vi "Estimate Mecanum Steering Frame.vi"(8 "error in (no error)":errorcluster, 11 "steering frame in":refnum<class "NI_Robotics_Steering Frame.lvclass">) -> (0 "error out":errorcluster, 2 "estimated mecanum steering frame copy":refnum<class "NI_Robotics_Mecanum Steering Frame.lvclass">, 3 "steering frame out":refnum<class "NI_Robotics_Steering Frame.lvclass">)   [LabVIEW 2017, in "NI_Robotics_Configure Steering Frame.lvlib"]
uses:
  <vilib>/robotics/Dialog/Configure Steering Frame/NI_Robotics_Configure Steering Frame.lvlib
  <vilib>/robotics/Steering/Steering Frame/NI_Robotics_Steering Frame.lvclass
  <vilib>/robotics/Steering/Mecanum Steering Frame/NI_Robotics_Mecanum Steering Frame.lvclass
  <vilib>/robotics/Steering/Steering Frame/NI_Robotics_Steering Frame.lvclass/NI_Robotics_Steering Frame.ctl
  <vilib>/robotics/Steering/Wheel/Wheel Parameters.ctl
  <vilib>/robotics/Steering/Wheel/Rotation Direction.ctl
  <vilib>/robotics/Steering/Mecanum Wheel/NI_Robotics_Mecanum Wheel.lvclass
  c:/Program Files (x86)/National Instruments/LabVIEW 2017/vi.lib/robotics/Steering/Wheel/NI_Robotics_Wheel.lvclass
  <vilib>/robotics/Steering/Wheel/NI_Robotics_Wheel.lvclass/NI_Robotics_Wheel.ctl
  <vilib>/robotics/Steering/Steering Frame/Get Multiple Wheels in Steering Frame.vi
  <vilib>/robotics/Steering/Wheel/Get General Wheel Information.vi
  <vilib>/robotics/Steering/Wheel/Get Wheel Radius.vi
  <vilib>/robotics/Steering/Wheel/Get Motor Communication.vi
  <vilib>/robotics/Steering/Wheel/Get Wheel Parameters.vi
  <vilib>/robotics/Steering/Mecanum Steering Frame/Create Mecanum Steering Frame.vi
  <vilib>/robotics/Steering/Omnidirectional Wheel/Create Omnidirectional Wheel.vi
  <vilib>/robotics/Steering/Mecanum Wheel/Create Mecanum Wheel.vi
  <vilib>/robotics/Steering/Caster Wheel/Create Caster Wheel.vi
  <vilib>/robotics/Steering/Steering Wheel/Create Steering Wheel.vi
  <vilib>/robotics/Steering/Fixed Wheel/Create Fixed Wheel.vi
  <vilib>/robotics/Steering/Wheel/NI_Robotics_Wheel.lvclass
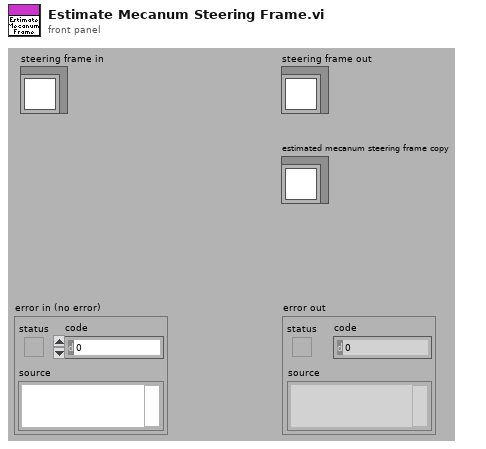
[diagram p1: front panel]
types:
  T1 = typedef "NI_Robotics_Wheel.lvclass/Wheel Parameters.ctl" = cluster{"wheel radius":dbl, "gear ratio":dbl, "forward rotation direction":T2}
  T2 = typedef "NI_Robotics_Wheel.lvclass/Rotation Direction.ctl" = u16
  T3 = cluster{"[0]":refnum<class "NI_Robotics_Mecanum Wheel.lvclass">, "[1]":refnum<class "NI_Robotics_Mecanum Wheel.lvclass">, "[2]":refnum<class "NI_Robotics_Mecanum Wheel.lvclass">, "[3]":refnum<class "NI_Robotics_Mecanum Wheel.lvclass">}
  T4 = cluster{"NI_Robotics_Mecanum Wheel.lvclass":refnum<class "NI_Robotics_Mecanum Wheel.lvclass">, "NI_Robotics_Mecanum Wheel.lvclass":refnum<class "NI_Robotics_Mecanum Wheel.lvclass">, "NI_Robotics_Mecanum Wheel.lvclass":refnum<class "NI_Robotics_Mecanum Wheel.lvclass">, "NI_Robotics_Mecanum Wheel.lvclass":refnum<class "NI_Robotics_Mecanum Wheel.lvclass">}
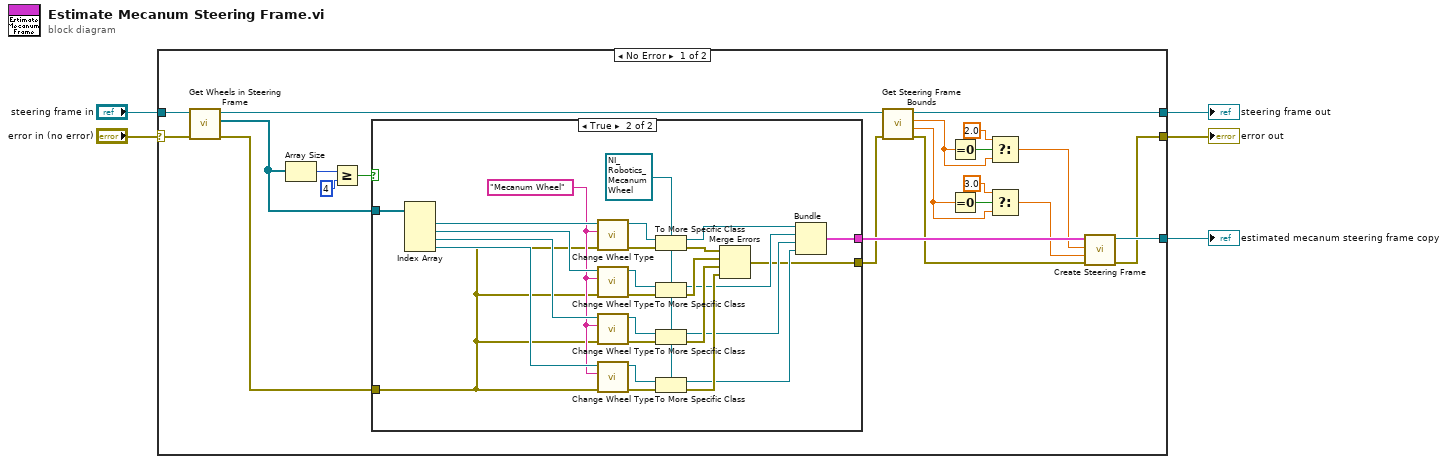
[diagram p0: block diagram]
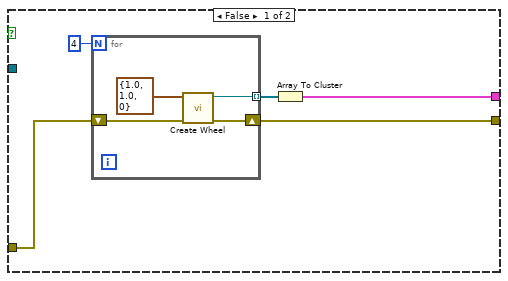
[diagram p2: hidden frame]
diagram:
  n1 = case shown="No Error" "error in (no error)" {
    selector: "error in (no error)" -> [w27 w64]
    tunnel: [w24 w64] -> w4
    tunnel: "steering frame in" -> [w26 w63]
    tunnel: [w17 w63] -> w2
    tunnel: [w25 _] -> w1
    frame No Error {
      n2 = call-poly <vilib>:"Get Wheels in Steering Frame.vi"("error in (no error)"=w27, "steering frame in"=w26) -> ("error out"=w19:errorcluster, "wheels"=w20:refnum<class "NI_Robotics_Wheel.lvclass">[], "steering frame out"=w6:refnum<class "NI_Robotics_Steering Frame.lvclass">)  [unwired: 3 in, 4 out]
      n3 = Array Size(array=w20) -> (size(s)=w23:i32)
      n4 = Greater Or Equal?(x=w23, y=4) -> (x >= y?=w21:bool)
      n5 = case shown="True" w21 {
        tunnel: w20 -> [_ w60]
        tunnel: w19 -> [w30 w37]
        tunnel: [w28 w41] -> w18
        tunnel: [w32 w40] -> w7
        frame False {
          n6 = for {
            N: 4 -> [_]
            shift-right: [w35] -> w32
            shift-left: w30 -> [w36]
            tunnel: [w34] -> w29 mode=indexing
            n7 = call-poly <vilib>:"Create Wheel.vi"("error in (no error)"=w36, "wheel parameters"=T1 {"wheel radius"=1.0, "gear ratio"=1.0, "forward rotation direction"=0}) -> ("error out"=w35:errorcluster, "mecanum wheel out"=w34:refnum<class "NI_Robotics_Mecanum Wheel.lvclass">)  [unwired: 8 in]
          }
          n8 = Array To Cluster(array=w29) -> (cluster=w28:T3)
        }
        frame True {
          w38 = refnum<class "NI_Robotics_Mecanum Wheel.lvclass"> refnum ("NI_Robotics_Mecanum Wheel.lvclass")
          w39 = "Mecanum Wheel" ("wheel type")
          n9 = Index Array(array=w60) -> (element #1=w59:refnum<class "NI_Robotics_Wheel.lvclass">, element #2=w55:refnum<class "NI_Robotics_Wheel.lvclass">, element #3=w54:refnum<class "NI_Robotics_Wheel.lvclass">, element #4=w53:refnum<class "NI_Robotics_Wheel.lvclass">)  [unwired: 4 in]
          n10 = call <vilib>:"Change Wheel Type.vi"("error in (no error)"=w37, "wheel type"=w39, "wheel in"=w59) -> ("error out"=w62:errorcluster, "wheel out"=w61:refnum<class "NI_Robotics_Wheel.lvclass">)  [unwired: 6 in, 1 out]
          n11 = call <vilib>:"Change Wheel Type.vi"("error in (no error)"=w37, "wheel type"=w39, "wheel in"=w55) -> ("error out"=w58:errorcluster, "wheel out"=w52:refnum<class "NI_Robotics_Wheel.lvclass">)  [unwired: 6 in, 1 out]
          n12 = call <vilib>:"Change Wheel Type.vi"("error in (no error)"=w37, "wheel type"=w39, "wheel in"=w54) -> ("error out"=w57:errorcluster, "wheel out"=w48:refnum<class "NI_Robotics_Wheel.lvclass">)  [unwired: 6 in, 1 out]
          n13 = call <vilib>:"Change Wheel Type.vi"("error in (no error)"=w37, "wheel type"=w39, "wheel in"=w53) -> ("error out"=w56:errorcluster, "wheel out"=w47:refnum<class "NI_Robotics_Wheel.lvclass">)  [unwired: 6 in, 1 out]
          n14 = To More Specific Class(target class=w38, reference=w61, error in=w62) -> (specific class reference=w45:refnum<class "NI_Robotics_Mecanum Wheel.lvclass">, error out=w51:errorcluster)
          n15 = To More Specific Class(target class=w38, reference=w52, error in=w58) -> (specific class reference=w44:refnum<class "NI_Robotics_Mecanum Wheel.lvclass">, error out=w50:errorcluster)
          n16 = To More Specific Class(target class=w38, reference=w48, error in=w57) -> (specific class reference=w43:refnum<class "NI_Robotics_Mecanum Wheel.lvclass">, error out=w49:errorcluster)
          n17 = To More Specific Class(target class=w38, reference=w47, error in=w56) -> (specific class reference=w42:refnum<class "NI_Robotics_Mecanum Wheel.lvclass">, error out=w46:errorcluster)
          n18 = Merge Errors(w51, w50, w49, w46) -> (w40:errorcluster)
          n19 = Bundle("NI_Robotics_Mecanum Wheel.lvclass"=w45, "NI_Robotics_Mecanum Wheel.lvclass"=w44, "NI_Robotics_Mecanum Wheel.lvclass"=w43, "NI_Robotics_Mecanum Wheel.lvclass"=w42) -> (w41:T4)  [unwired: 1 in]
        }
      }
      n20 = call <vilib>:"Get Steering Frame Bounds.vi"("error in (no error)"=w7, "steering frame in"=w6) -> ("error out"=w8:errorcluster, "length"=w10:dbl, "width"=w15:dbl, "steering frame out"=w17:refnum<class "NI_Robotics_Steering Frame.lvclass">)  [unwired: 4 in, 2 out]
      n21 = Equal To 0?(x=w15) -> (x = 0?=w16:bool)
      n22 = Equal To 0?(x=w10) -> (x = 0?=w12:bool)
      n23 = Select(t=2.0 ("wheel separation"), s=w16, f=w15) -> (s? t:f=w14:dbl)
      n24 = Select(t=3.0 ("wheel separation"), s=w12, f=w10) -> (s? t:f=w9:dbl)
      n25 = call-poly <vilib>:"Create Steering Frame.vi"("error in (no error)"=w8, "wheel separation length"=w9, "wheel separation width"=w14, "wheels"=w18) -> ("error out"=w24:errorcluster, "mecanum steering frame out"=w25:refnum<class "NI_Robotics_Mecanum Steering Frame.lvclass">)  [unwired: 6 in]
    }
    frame Error {
    }
  }
  "steering frame out" <- w2
  "error out" <- w4
  "estimated mecanum steering frame copy" <- w1
